vi "st_Poisson PDF (kx).vi"(10 "a":dbl=0.5, 11 "x":dbl=1.0) -> (0 "error":i32, 3 "pdf(x)":dbl=0.3032653298563167)   [LabVIEW 2024, in "NI_Gmath.lvlib"]
uses:
  NI_Gmath.lvlib
  st_error_code.ctl
panel:
  # "Poisson PDF"
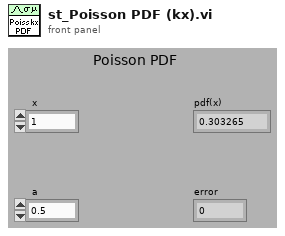
[diagram p1: front panel]
types:
  T1 = typedef "NI_Gmath.lvlib/st_error_code.ctl" = i32
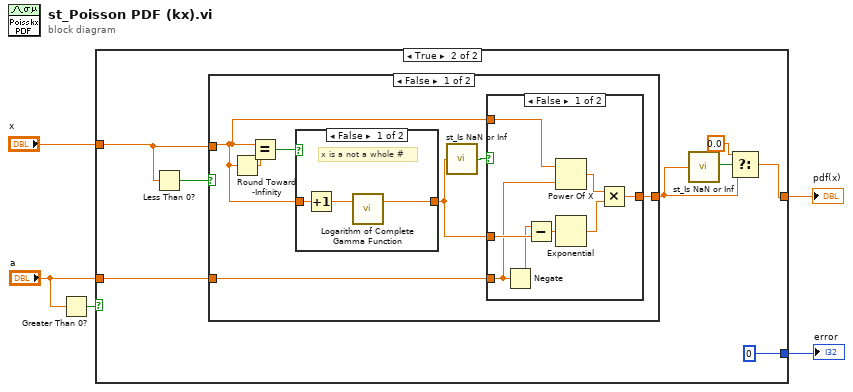
[diagram p0: block diagram]
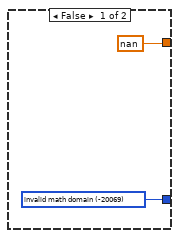
[diagram p2: hidden frame]
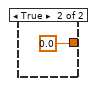
[diagram p3: hidden frame]
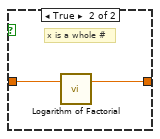
[diagram p4: hidden frame]
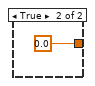
[diagram p5: hidden frame]
diagram:
  n1 = Greater Than 0?(x="a") -> (x > 0?=w1:bool)
  n2 = case shown="True" w1 {
    tunnel: [w6 0 ("invalid math domain")] -> w5
    tunnel: [nan w10] -> w4
    tunnel: "x" -> [_ w12]
    tunnel: "a" -> [_ w13]
    frame False {
      w6 = T1 -20069 items=["invalid math domain"=-20069, "Fourier interpolation size m >= n"=-20070, "empty array"=-20003] ("stat interp error code")
    }
    frame True {
      n3 = Less Than 0?(x=w12) -> (x < 0?=w14:bool)
      n4 = case shown="False" w14 {
        tunnel: [w19 0.0] -> w9
        tunnel: w13 -> [w17 _]
        tunnel: w12 -> [w16 _]
        frame False {
          n5 = Round Toward -Infinity(1:w16) -> (0:w22:dbl)
          n6 = Equal?(x=w16, y=w22) -> (x = y?=w21:bool)
          n7 = case shown="False" w21 {
            tunnel: w16 -> [w34 w36]
            tunnel: [w32 w35] -> w18
            frame False {
              # "x is a not a whole #"
              n8 = Increment(x=w34) -> (x+1=w33:dbl)
              n9 = call "Logarithm of Complete Gamma Function.vi"("x"=w33) -> ("ln(g(x))"=w32:dbl)  [unwired: 2 in]
            }
            frame True {
              # "x is a whole #"
              n10 = call "Logarithm of Factorial.vi"("n"=w36) -> ("ln(n!)"=w35:dbl)  [unwired: 2 in]
            }
          }
          n11 = call "st_Is NaN or Inf.vi"("x"=w18) -> ("isNaN(x) || isInf(x)"=w20:bool)  [unwired: 4 in]
          n12 = case shown="False" w20 {
            tunnel: [w23 0.0] -> w19
            tunnel: w18 -> [w30 _]
            tunnel: w17 -> [w25 _]
            tunnel: w16 -> [w24 _]
            frame False {
              n13 = Negate(x=w25) -> (-x=w29:dbl)
              n14 = Subtract(x=w29, y=w30) -> (x-y=w28:dbl)
              n15 = Power Of X(1:w25, 2:w24) -> (0:w27:dbl)
              n16 = Exponential(1:w28) -> (0:w26:dbl)
              n17 = Multiply(x=w27, y=w26) -> (x*y=w23:dbl)
            }
            frame True {
            }
          }
        }
        frame True {
        }
      }
      n18 = call "st_Is NaN or Inf.vi"("x"=w9) -> ("isNaN(x) || isInf(x)"=w8:bool)  [unwired: 4 in]
      n19 = Select(t=0.0, s=w8, f=w9) -> (s? t:f=w10:dbl)
    }
  }
  "pdf(x)" <- w4
  "error" <- w5
